vi "Login.vi"(0 "User Manager View in":refnum<class "User Manager View.lvclass">, 5 "User Login Information":T1, 11 "error in (no error)":errorcluster) -> (4 "User Manager View out":refnum<class "User Manager View.lvclass">, 15 "error out":errorcluster)   [LabVIEW 2017, in "User Manager View.lvlib" / "User Manager View.lvclass"]
uses:
  <vilib>/gpm_packages/@cs/User Manager App/User Manager View/User Manager View/User Manager View.lvclass
  <vilib>/gpm_packages/@cs/User Manager App/User Manager Model/Type Definitions/Successful Login Information.ctl
  <vilib>/gpm_packages/@cs/User Manager App/User Manager Model/Type Definitions/User Levels.ctl
  <vilib>/gpm_packages/@cs/User Manager App/User Manager View/User Manager View/User Manager View.lvclass/User Manager View.ctl
  <vilib>/gpm_packages/@cs/User Manager App/User Manager Model/Type Definitions/User Manager Application Types.lvlib
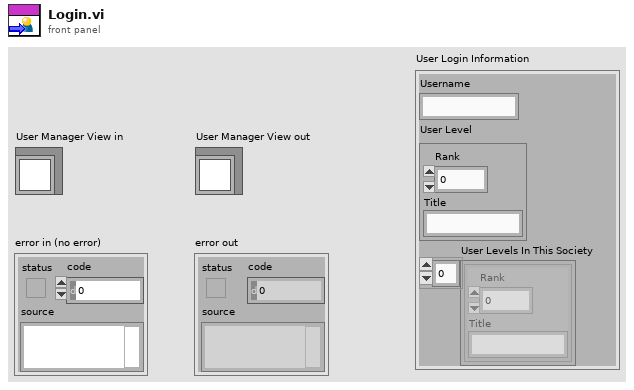
[diagram p1: front panel]
types:
  T1 = typedef "User Manager Application Types.lvlib/Successful Login Information.ctl" = cluster{"Username":string, "User Level":T2, "User Levels In This Society":T2[]}
  T2 = typedef "User Manager Application Types.lvlib/User Levels.ctl" = cluster{"Rank":i32, "Title":string}
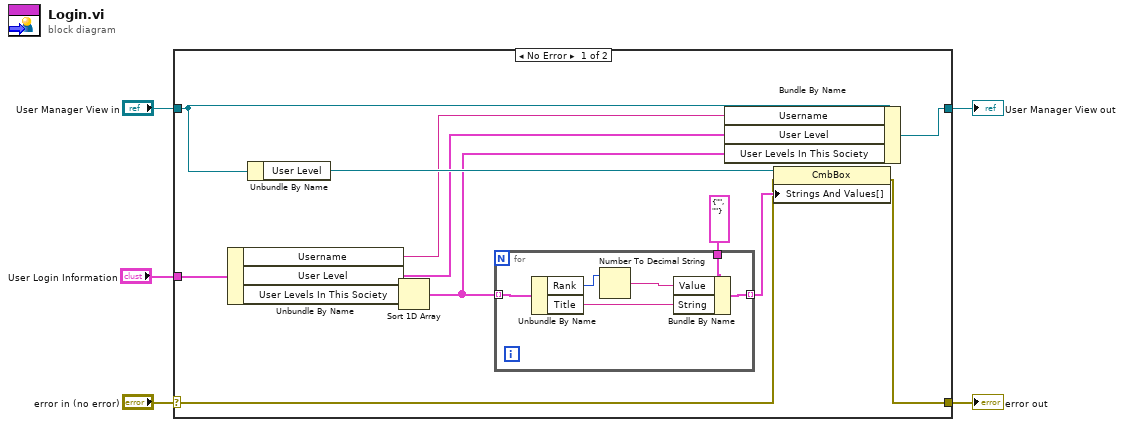
[diagram p0: block diagram]
diagram:
  n1 = case shown="No Error" "error in (no error)" {
    selector: "error in (no error)" -> [w6 w25]
    tunnel: [w9 w25] -> w4
    tunnel: [w16 w24] -> w2
    tunnel: "User Manager View in" -> [w17 w24]
    tunnel: "User Login Information" -> [w12 _]
    frame No Error {
      n2 = Unbundle By Name(w12) -> ("Username"=w8:string, "User Level"=w7:T2, "User Levels In This Society"=w11:T2[])
      n3 = Unbundle By Name(w17) -> ("User Level"=w13:refnum<vi>)
      n4 = Sort 1D Array(array=w11) -> (sorted array=w10:T2[])
      n5 = for {
        tunnel: cluster{"String":string, "Value":string} {"String"="", "Value"=""} -> [w23]
        tunnel: w10 -> [w21] mode=indexing
        tunnel: [w22] -> w14 mode=indexing
        n6 = Unbundle By Name(w21) -> ("Rank"=w18:i32, "Title"=w19:string)
        n7 = Number To Decimal String(number=w18) -> (decimal integer string=w20:string)  [unwired: 1 in]
        n8 = Bundle By Name(cluster=w23, "Value"=w20, "String"=w19) -> (w22:cluster{"String":string, "Value":string})
      }
      n9 = Bundle By Name(cluster=w17, "Username"=w8, "User Level"=w7, "User Levels In This Society"=w10) -> (w16:refnum<class "User Manager View.lvclass">)
      n10 = property class="CmbBox"(reference=w13, error in=w6, "Strings And Values[]"=w14) -> (error out=w9:errorcluster)  [unwired: 1 out]
    }
    frame Error {
    }
  }
  "error out" <- w4
  "User Manager View out" <- w2
